vi "Persist Entity.vi"(8 "error in (no error)":errorcluster, 9 "Conditum:Entity":refnum<class "Entity.lvclass">, 10 "Types":refnum<class "Type.lvclass">[](array[class]), 11 "Database in":refnum<class "Database Platform.lvclass">) -> (0 "error out":errorcluster, 3 "Database out":refnum<class "Database Platform.lvclass">)   [LabVIEW 2020, in "Conditu2.lvlib" / "Database Platform.lvclass"]
uses:
  Database Platform.lvclass
  Entity/Entity.lvclass
  Columns/Type/Type.lvclass
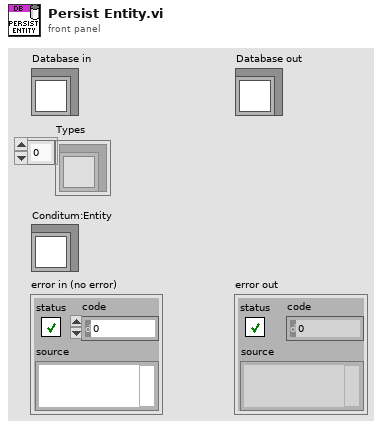
[diagram p1: front panel]
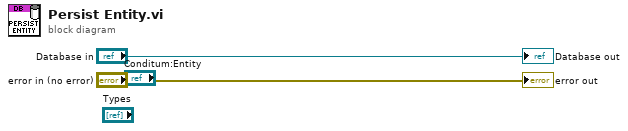
[diagram p0: block diagram]
diagram:
  "error out" <- "error in (no error)"
  "Database out" <- "Database in"
